vi "Stop Core.vi"(10 "final error code":i32, 11 "Manager in":refnum<class "Manager.lvclass">) -> (3 "Manager out":refnum<class "Manager.lvclass">)   [LabVIEW 2013, in "Manager.lvlib" / "Manager.lvclass"]
uses:
  Manager.lvclass
  PluginInterface/Actor Framework.lvlibp/Actor/Actor.lvclass
  Manager.lvclass/Manager.ctl
  Read Control Systems.vi
  PluginInterface/Actor Framework.lvlibp/Stop Msg/Stop Msg.lvclass
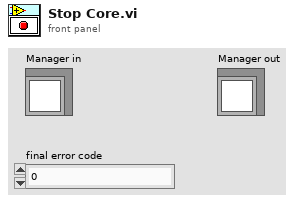
[diagram p1: front panel]
types:
  T1 = cluster{"Name":string, "Plugins":refnum<class "Message Enqueuer.lvclass">[]}[]
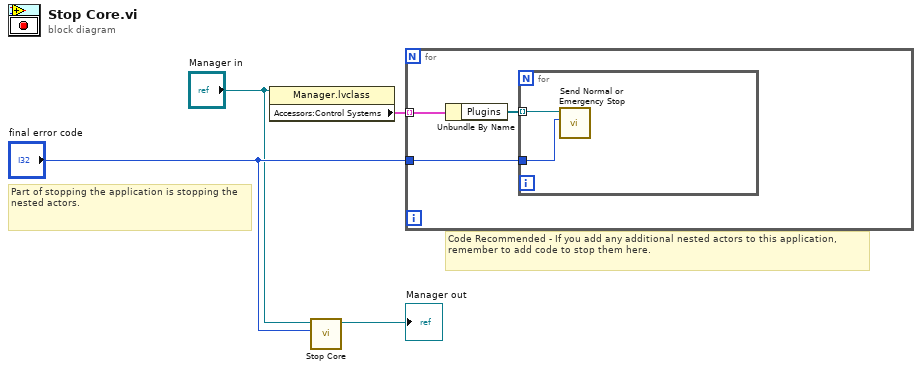
[diagram p0: block diagram]
diagram:
  # "Code Recommended - If you add any additional nested actors to this application, remember to add code to stop them here."
  # "Part of stopping the application is stopping the nested actors."
  n1 = property class="Manager.lvclass"(reference="Manager in") -> ("Accessors:Control Systems"=w1:T1)  [unwired: 1 in, 2 out]
  n2 = call-parent "Stop Core.vi"("final error code"="final error code", "Actor in"="Manager in") -> ("Actor out"=→"Manager out":refnum<class "Manager.lvclass">)  [unwired: 9 in]
  n3 = for {
    tunnel: "final error code" -> [w6]
    tunnel: w1 -> [w7] mode=indexing
    n4 = Unbundle By Name(w7) -> ("Plugins"=w5:refnum<class "Message Enqueuer.lvclass">[])
    n5 = for {
      tunnel: w5 -> [w9] mode=indexing
      tunnel: w6 -> [w8]
      n6 = call "Send Normal or Emergency Stop.vi"("final error code"=w8, "Message Enqueuer"=w9) -> ()  [unwired: 9 in, 1 out]
    }
  }
